vi "GOOP_GetDefaultInstance.vi"(8 "error in":errorcluster, 11 "LVClassIn":refnum<vi>) -> (0 "error out":errorcluster, 2 "ClassWriter.lvclass":refnum<class "ClassWriter.lvclass">, 3 "LVClassOut":refnum<vi>)   [LabVIEW 2016]
uses:
  <resource>/Framework/Providers/Open_GDS/ClassProviders/Provider_BaseClassInterface/ClassWriter_class/ClassWriter.lvclass
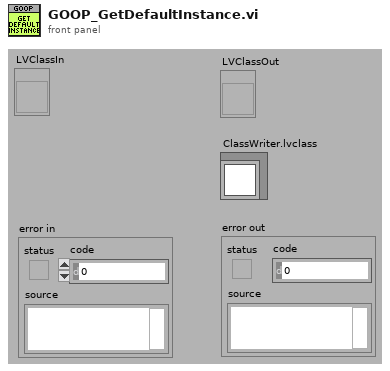
[diagram p1: front panel]
types:
  T1 = cluster{"Major":u16, "Minor":u16, "Fix":u16, "Build":u16}
  T2 = cluster{"Path":path, "Version":cluster{"Major":u16, "Minor":u16, "Fix":u16, "Build":u16}, "App.Version":string, "App.UserName":string}
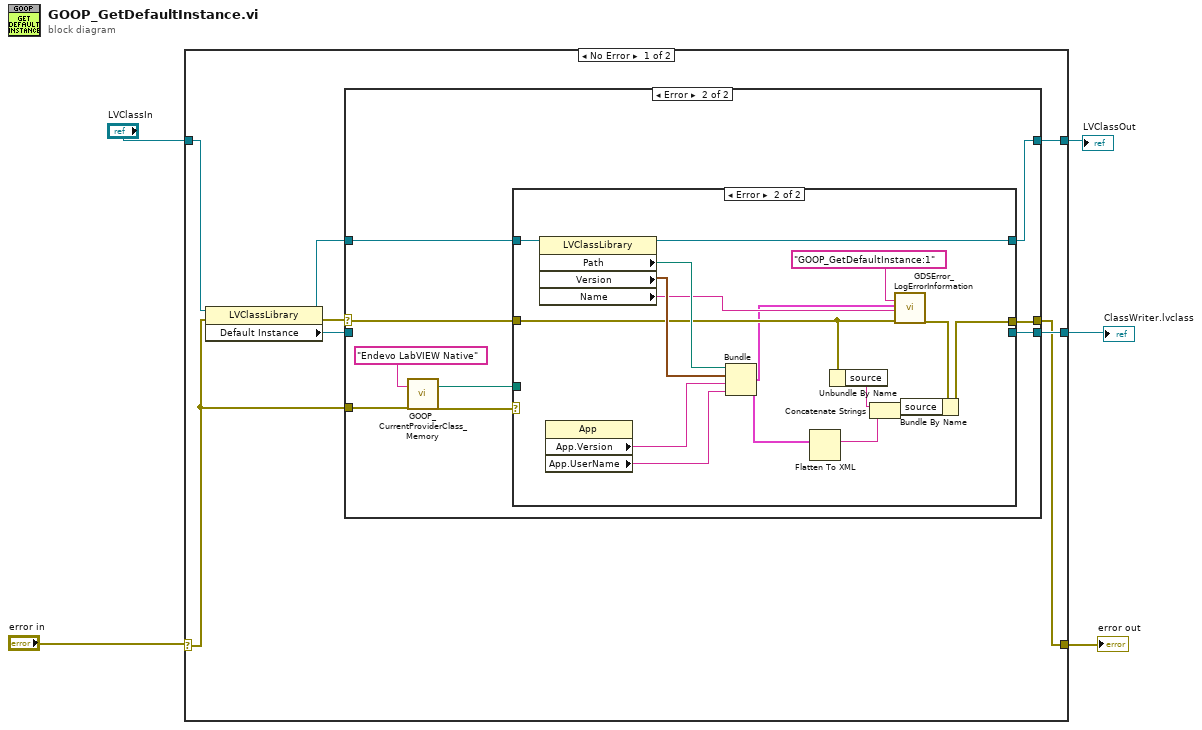
[diagram p0: block diagram]
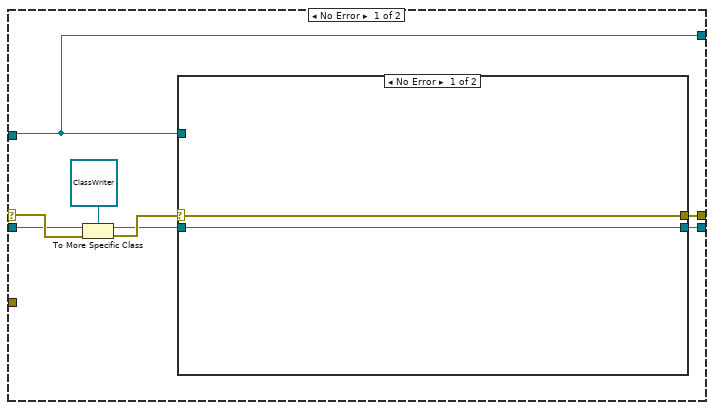
[diagram p2: hidden frame]
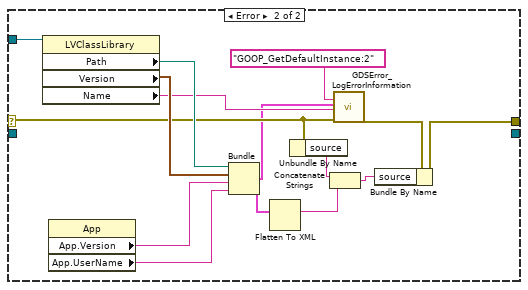
[diagram p3: hidden frame]
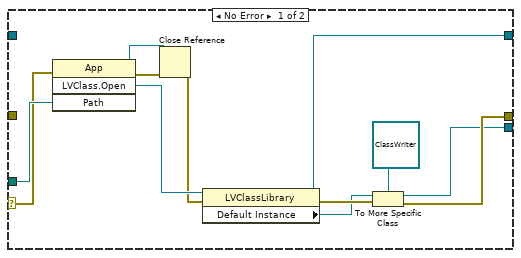
[diagram p4: hidden frame]
diagram:
  n1 = case shown="No Error" "error in" {
    selector: "error in" -> [w7 w74]
    tunnel: [w9 w74] -> w5
    tunnel: [w6 w75] -> w4
    tunnel: "LVClassIn" -> [w13 w75]
    tunnel: [w11 _] -> w1
    frame No Error {
      n2 = property class="LVClassLibrary"(reference=w13, error in=w7) -> (reference out=w8:refnum<vi>, error out=w10:errorcluster, "Default Instance"=w12:refnum<class>)
      n3 = case shown="Error" w10 {
        selector: w10 -> [w20 w45]
        tunnel: [w17 w44] -> w9
        tunnel: w12 -> [w19 _]
        tunnel: [w15 w38] -> w11
        tunnel: w8 -> [w14 w46]
        tunnel: w7 -> [_ w42]
        tunnel: [w14 w39] -> w6
        frame No Error {
          n4 = To More Specific Class(target class=refnum<class "ClassWriter.lvclass"> refnum ("ClassWriter.lvclass"), reference=w19, error in=w20) -> (specific class reference=w16:refnum<class "ClassWriter.lvclass">, error out=w18:errorcluster)
          n5 = case shown="No Error" w18 {
            selector: w18 -> [w23 w28]
            tunnel: [w23 w29] -> w17
            tunnel: w16 -> [w22 _]
            tunnel: [w22 _] -> w15
            tunnel: w14 -> [_ w31]
            frame No Error {
            }
            frame Error {
              n6 = property class="LVClassLibrary"(reference=w31) -> ("Path"=w36:path, "Version"=w35:T1, "Name"=w32:string)  [unwired: 1 in, 2 out]
              n7 = property class="App"() -> ("App.Version"=w34:string, "App.UserName"=w33:string)  [unwired: 2 in, 2 out]
              n8 = Bundle("Path"=w36, "Version"=w35, "App.Version"=w34, "App.UserName"=w33) -> (w25:T2)  [unwired: 1 in]
              n9 = Flatten To XML(anything=w25) -> (xml string=w24:string)
              n10 = Unbundle By Name(w28) -> ("source"=w27:string)
              n11 = Concatenate Strings(w27, w24) -> (w26:string)
              n12 = call <resource>:"GDSError_LogErrorInformation.vi"("State"="GOOP_GetDefaultInstance:2", "LocalVariableData"=w25, "ExtraErrorInfo"=w32, "error in (no error)"=w28) -> ("error out"=w30:errorcluster)  [unwired: 15 in]
              n13 = Bundle By Name(cluster=w30, "source"=w26) -> (w29:errorcluster)
            }
          }
        }
        frame Error {
          n14 = call <resource>:"GOOP_CurrentProviderClass_Memory.vi"("GetThisClassProvidersPaths(Returns the default providor if not wired)"="Endevo LabVIEW Native", "error in (no error)"=w42) -> ("ClassProviderClassWriterPath"=w40:path, "error out"=w41:errorcluster)  [unwired: 13 in, 3 out]
          n15 = case shown="Error" w41 {
            selector: w41 -> [w55 _]
            tunnel: w46 -> [_ w72]
            tunnel: w45 -> [_ w63]
            tunnel: [w49 w61] -> w44
            tunnel: w40 -> [w56 _]
            tunnel: [w48 w59] -> w39
            tunnel: [w47 _] -> w38
            frame No Error {
              n16 = invoke class="App" method="LVClass.Open"(error in=w55, "Path"=w56) -> (reference out=w57:refnum<vi>, error out=w54:errorcluster, "LVClass.Open"=w53:refnum<vi>)  [unwired: 2 in, 1 out]
              n17 = Close Reference(reference=w57, error in (no error)=w54) -> (error out=w50:errorcluster)
              n18 = property class="LVClassLibrary"(reference=w53, error in=w50) -> (reference out=w48:refnum<vi>, error out=w52:errorcluster, "Default Instance"=w51:refnum<class>)
              n19 = To More Specific Class(target class=refnum<class "ClassWriter.lvclass"> refnum ("ClassWriter.lvclass"), reference=w51, error in=w52) -> (specific class reference=w47:refnum<class "ClassWriter.lvclass">, error out=w49:errorcluster)
            }
            frame Error {
              n20 = property class="LVClassLibrary"(reference=w72) -> (reference out=w59:refnum<vi>, "Path"=w71:path, "Version"=w70:T1, "Name"=w67:string)  [unwired: 1 in, 1 out]
              n21 = property class="App"() -> ("App.Version"=w69:string, "App.UserName"=w68:string)  [unwired: 2 in, 2 out]
              n22 = Bundle("Path"=w71, "Version"=w70, "App.Version"=w69, "App.UserName"=w68) -> (w60:T2)  [unwired: 1 in]
              n23 = Flatten To XML(anything=w60) -> (xml string=w64:string)
              n24 = Unbundle By Name(w63) -> ("source"=w66:string)
              n25 = Concatenate Strings(w66, w64) -> (w65:string)
              n26 = call <resource>:"GDSError_LogErrorInformation.vi"("State"="GOOP_GetDefaultInstance:1", "LocalVariableData"=w60, "ExtraErrorInfo"=w67, "error in (no error)"=w63) -> ("error out"=w62:errorcluster)  [unwired: 15 in]
              n27 = Bundle By Name(cluster=w62, "source"=w65) -> (w61:errorcluster)
            }
          }
        }
      }
    }
    frame Error {
    }
  }
  "error out" <- w5
  "LVClassOut" <- w4
  "ClassWriter.lvclass" <- w1
